vi "latchSignalsForConfiguredTime.vi"(8 "error in (no error)":errorcluster, 11 "cRIOScanModeTarget in":refnum<class "cRIOScanModeTarget.lvclass">) -> (0 "error out":errorcluster, 3 "cRIOScanModeTarget out":refnum<class "cRIOScanModeTarget.lvclass">)   [LabVIEW 2012, in "cRIOScanModeTarget.lvclass"]
uses:
  cRIOScanModeTarget.lvclass
  cRIOScanModeTarget.lvclass/cRIOScanModeTarget.ctl
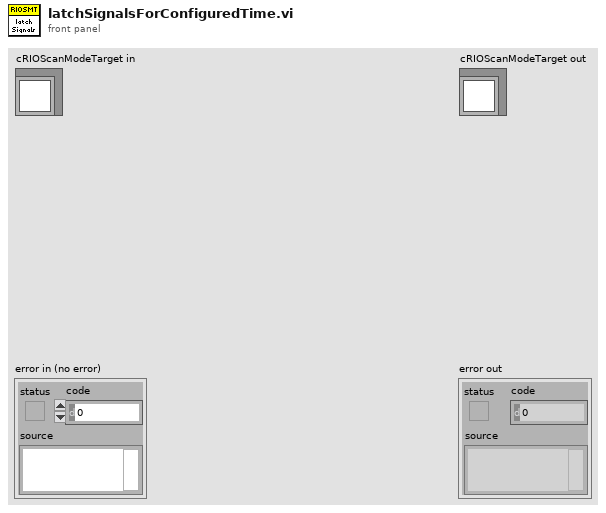
[diagram p1: front panel]
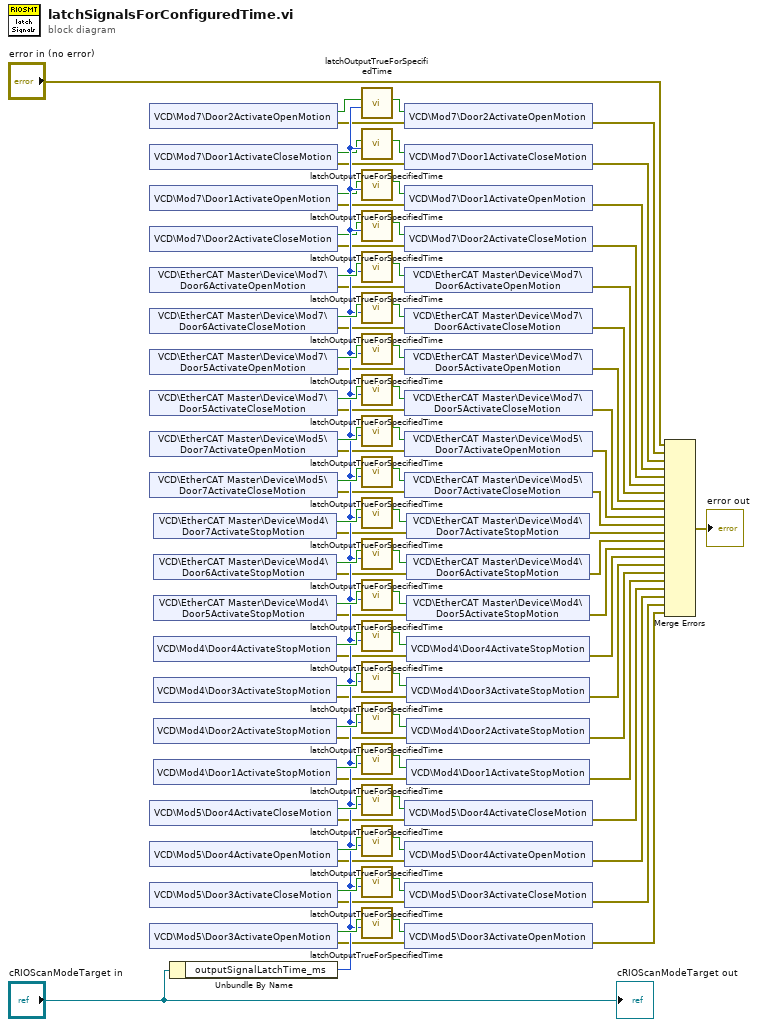
[diagram p0: block diagram]
diagram:
  n1 = shared-variable "VCD\\Mod7\\Door2ActivateOpenMotion"() -> (w44:bool, error out=w22:errorcluster)  [unwired: 1 in]
  n2 = shared-variable "VCD\\Mod7\\Door1ActivateCloseMotion"() -> (w45:bool, error out=w23:errorcluster)  [unwired: 1 in]
  n3 = shared-variable "VCD\\Mod7\\Door1ActivateOpenMotion"() -> (w46:bool, error out=w24:errorcluster)  [unwired: 1 in]
  n4 = shared-variable "VCD\\Mod7\\Door2ActivateCloseMotion"() -> (w43:bool, error out=w25:errorcluster)  [unwired: 1 in]
  n5 = shared-variable "VCD\\EtherCAT Master\\Device\\Mod7\\Door6ActivateOpenMotion"() -> (w82:bool, error out=w26:errorcluster)  [unwired: 1 in]
  n6 = shared-variable "VCD\\EtherCAT Master\\Device\\Mod7\\Door6ActivateCloseMotion"() -> (w83:bool, error out=w27:errorcluster)  [unwired: 1 in]
  n7 = shared-variable "VCD\\EtherCAT Master\\Device\\Mod7\\Door5ActivateOpenMotion"() -> (w84:bool, error out=w28:errorcluster)  [unwired: 1 in]
  n8 = shared-variable "VCD\\EtherCAT Master\\Device\\Mod7\\Door5ActivateCloseMotion"() -> (w85:bool, error out=w29:errorcluster)  [unwired: 1 in]
  n9 = shared-variable "VCD\\EtherCAT Master\\Device\\Mod5\\Door7ActivateOpenMotion"() -> (w76:bool, error out=w30:errorcluster)  [unwired: 1 in]
  n10 = shared-variable "VCD\\EtherCAT Master\\Device\\Mod5\\Door7ActivateCloseMotion"() -> (w77:bool, error out=w31:errorcluster)  [unwired: 1 in]
  n11 = shared-variable "VCD\\Mod5\\Door4ActivateCloseMotion"() -> (w59:bool, error out=w39:errorcluster)  [unwired: 1 in]
  n12 = shared-variable "VCD\\Mod5\\Door4ActivateOpenMotion"() -> (w58:bool, error out=w40:errorcluster)  [unwired: 1 in]
  n13 = shared-variable "VCD\\Mod5\\Door3ActivateCloseMotion"() -> (w57:bool, error out=w41:errorcluster)  [unwired: 1 in]
  n14 = shared-variable "VCD\\Mod5\\Door3ActivateOpenMotion"() -> (w56:bool, error out=w42:errorcluster)  [unwired: 1 in]
  n15 = shared-variable "VCD\\EtherCAT Master\\Device\\Mod4\\Door7ActivateStopMotion"() -> (w73:bool, error out=w32:errorcluster)  [unwired: 1 in]
  n16 = shared-variable "VCD\\EtherCAT Master\\Device\\Mod4\\Door6ActivateStopMotion"() -> (w72:bool, error out=w33:errorcluster)  [unwired: 1 in]
  n17 = shared-variable "VCD\\EtherCAT Master\\Device\\Mod4\\Door5ActivateStopMotion"() -> (w71:bool, error out=w34:errorcluster)  [unwired: 1 in]
  n18 = shared-variable "VCD\\Mod4\\Door4ActivateStopMotion"() -> (w60:bool, error out=w35:errorcluster)  [unwired: 1 in]
  n19 = shared-variable "VCD\\Mod4\\Door3ActivateStopMotion"() -> (w61:bool, error out=w36:errorcluster)  [unwired: 1 in]
  n20 = shared-variable "VCD\\Mod4\\Door2ActivateStopMotion"() -> (w62:bool, error out=w37:errorcluster)  [unwired: 1 in]
  n21 = shared-variable "VCD\\Mod4\\Door1ActivateStopMotion"() -> (w63:bool, error out=w38:errorcluster)  [unwired: 1 in]
  n22 = Unbundle By Name("cRIOScanModeTarget in") -> ("outputSignalLatchTime_ms"=w51:u32)
  n23 = call <userlib>:"latchOutputTrueForSpecifiedTime.vi"("latchTime_ms"=w51, "Value"=w44) -> ("outputValue"=w49:bool)  [unwired: 9 in]
  n24 = call <userlib>:"latchOutputTrueForSpecifiedTime.vi"("latchTime_ms"=w51, "Value"=w45) -> ("outputValue"=w48:bool)  [unwired: 9 in]
  n25 = call <userlib>:"latchOutputTrueForSpecifiedTime.vi"("latchTime_ms"=w51, "Value"=w46) -> ("outputValue"=w47:bool)  [unwired: 9 in]
  n26 = call <userlib>:"latchOutputTrueForSpecifiedTime.vi"("latchTime_ms"=w51, "Value"=w43) -> ("outputValue"=w50:bool)  [unwired: 9 in]
  n27 = call <userlib>:"latchOutputTrueForSpecifiedTime.vi"("latchTime_ms"=w51, "Value"=w82) -> ("outputValue"=w81:bool)  [unwired: 9 in]
  n28 = call <userlib>:"latchOutputTrueForSpecifiedTime.vi"("latchTime_ms"=w51, "Value"=w83) -> ("outputValue"=w80:bool)  [unwired: 9 in]
  n29 = call <userlib>:"latchOutputTrueForSpecifiedTime.vi"("latchTime_ms"=w51, "Value"=w84) -> ("outputValue"=w79:bool)  [unwired: 9 in]
  n30 = call <userlib>:"latchOutputTrueForSpecifiedTime.vi"("latchTime_ms"=w51, "Value"=w85) -> ("outputValue"=w78:bool)  [unwired: 9 in]
  n31 = call <userlib>:"latchOutputTrueForSpecifiedTime.vi"("latchTime_ms"=w51, "Value"=w76) -> ("outputValue"=w75:bool)  [unwired: 9 in]
  n32 = call <userlib>:"latchOutputTrueForSpecifiedTime.vi"("latchTime_ms"=w51, "Value"=w77) -> ("outputValue"=w74:bool)  [unwired: 9 in]
  n33 = call <userlib>:"latchOutputTrueForSpecifiedTime.vi"("latchTime_ms"=w51, "Value"=w73) -> ("outputValue"=w68:bool)  [unwired: 9 in]
  n34 = call <userlib>:"latchOutputTrueForSpecifiedTime.vi"("latchTime_ms"=w51, "Value"=w72) -> ("outputValue"=w69:bool)  [unwired: 9 in]
  n35 = call <userlib>:"latchOutputTrueForSpecifiedTime.vi"("latchTime_ms"=w51, "Value"=w71) -> ("outputValue"=w70:bool)  [unwired: 9 in]
  n36 = call <userlib>:"latchOutputTrueForSpecifiedTime.vi"("latchTime_ms"=w51, "Value"=w60) -> ("outputValue"=w67:bool)  [unwired: 9 in]
  n37 = call <userlib>:"latchOutputTrueForSpecifiedTime.vi"("latchTime_ms"=w51, "Value"=w61) -> ("outputValue"=w66:bool)  [unwired: 9 in]
  n38 = call <userlib>:"latchOutputTrueForSpecifiedTime.vi"("latchTime_ms"=w51, "Value"=w62) -> ("outputValue"=w65:bool)  [unwired: 9 in]
  n39 = call <userlib>:"latchOutputTrueForSpecifiedTime.vi"("latchTime_ms"=w51, "Value"=w63) -> ("outputValue"=w64:bool)  [unwired: 9 in]
  n40 = call <userlib>:"latchOutputTrueForSpecifiedTime.vi"("latchTime_ms"=w51, "Value"=w59) -> ("outputValue"=w55:bool)  [unwired: 9 in]
  n41 = call <userlib>:"latchOutputTrueForSpecifiedTime.vi"("latchTime_ms"=w51, "Value"=w58) -> ("outputValue"=w54:bool)  [unwired: 9 in]
  n42 = call <userlib>:"latchOutputTrueForSpecifiedTime.vi"("latchTime_ms"=w51, "Value"=w57) -> ("outputValue"=w53:bool)  [unwired: 9 in]
  n43 = call <userlib>:"latchOutputTrueForSpecifiedTime.vi"("latchTime_ms"=w51, "Value"=w56) -> ("outputValue"=w52:bool)  [unwired: 9 in]
  n44 = shared-variable "VCD\\Mod7\\Door2ActivateOpenMotion"(w49, error in=w22) -> (error out=w21:errorcluster)
  n45 = shared-variable "VCD\\Mod7\\Door1ActivateCloseMotion"(w48, error in=w23) -> (error out=w20:errorcluster)
  n46 = shared-variable "VCD\\Mod7\\Door1ActivateOpenMotion"(w47, error in=w24) -> (error out=w19:errorcluster)
  n47 = shared-variable "VCD\\Mod7\\Door2ActivateCloseMotion"(w50, error in=w25) -> (error out=w18:errorcluster)
  n48 = shared-variable "VCD\\EtherCAT Master\\Device\\Mod7\\Door6ActivateOpenMotion"(w81, error in=w26) -> (error out=w17:errorcluster)
  n49 = shared-variable "VCD\\EtherCAT Master\\Device\\Mod7\\Door6ActivateCloseMotion"(w80, error in=w27) -> (error out=w16:errorcluster)
  n50 = shared-variable "VCD\\EtherCAT Master\\Device\\Mod7\\Door5ActivateOpenMotion"(w79, error in=w28) -> (error out=w15:errorcluster)
  n51 = shared-variable "VCD\\EtherCAT Master\\Device\\Mod7\\Door5ActivateCloseMotion"(w78, error in=w29) -> (error out=w14:errorcluster)
  n52 = shared-variable "VCD\\EtherCAT Master\\Device\\Mod5\\Door7ActivateOpenMotion"(w75, error in=w30) -> (error out=w13:errorcluster)
  n53 = shared-variable "VCD\\EtherCAT Master\\Device\\Mod5\\Door7ActivateCloseMotion"(w74, error in=w31) -> (error out=w12:errorcluster)
  n54 = shared-variable "VCD\\Mod5\\Door4ActivateCloseMotion"(w55, error in=w39) -> (error out=w4:errorcluster)
  n55 = shared-variable "VCD\\Mod5\\Door4ActivateOpenMotion"(w54, error in=w40) -> (error out=w3:errorcluster)
  n56 = shared-variable "VCD\\Mod5\\Door3ActivateCloseMotion"(w53, error in=w41) -> (error out=w2:errorcluster)
  n57 = shared-variable "VCD\\Mod5\\Door3ActivateOpenMotion"(w52, error in=w42) -> (error out=w1:errorcluster)
  n58 = shared-variable "VCD\\EtherCAT Master\\Device\\Mod4\\Door7ActivateStopMotion"(w68, error in=w32) -> (error out=w11:errorcluster)
  n59 = shared-variable "VCD\\EtherCAT Master\\Device\\Mod4\\Door6ActivateStopMotion"(w69, error in=w33) -> (error out=w10:errorcluster)
  n60 = shared-variable "VCD\\EtherCAT Master\\Device\\Mod4\\Door5ActivateStopMotion"(w70, error in=w34) -> (error out=w9:errorcluster)
  n61 = shared-variable "VCD\\Mod4\\Door4ActivateStopMotion"(w67, error in=w35) -> (error out=w8:errorcluster)
  n62 = shared-variable "VCD\\Mod4\\Door3ActivateStopMotion"(w66, error in=w36) -> (error out=w7:errorcluster)
  n63 = shared-variable "VCD\\Mod4\\Door2ActivateStopMotion"(w65, error in=w37) -> (error out=w6:errorcluster)
  n64 = shared-variable "VCD\\Mod4\\Door1ActivateStopMotion"(w64, error in=w38) -> (error out=w5:errorcluster)
  n65 = Merge Errors("error in (no error)", w21, w20, w19, w18, w17, w16, w15, w14, w13, w12, w11, w10, w9, w8, w7, w6, w5, w4, w3, w2, w1) -> (→"error out":errorcluster)
  "cRIOScanModeTarget out" <- "cRIOScanModeTarget in"
